vi "SmarAct micropositioner control.vi"() -> ()   [LabVIEW 2013]
uses:
  <vilib>/Utility/file.llb/Write To Spreadsheet File (DBL).vi
  <vilib>/DAQmx/configure/timing.llb/DAQmx Timing (Implicit).vi
  <vilib>/DAQmx/create/channels.llb/DAQmx Create Channel (CO-Pulse Generation-Frequency).vi
panel:
  in  "counter":tag="Dev1/ctr0" caption="计数器"
  out "frequency":dbl=1.0 format="%#_13g"
  out "duty cycle":dbl=0.5 caption="占空比" format="%.6f"
  in  "samples per channel":i32=5 caption="脉冲个数"
  in  "周期（ms）":dbl=1.0 format="%#_13g"
  in  "脉宽（us）":dbl=10.0 format="%#_13g"
  in  "initial delay":dbl format="%.6f"
  in  "X扫描步距":i16
  out "已完成行数":i32
  out "存储数据time,x,y":dbl[][](array[numeric])
  out "完成":bool
  out "error out":errorcluster
  in  "Y 初始位置":i32
  in  "X 初始位置":i32
  in  "X 返回速度":u32=50 min=1 max=4095000000
  out "error out 2":errorcluster
  out "XY 实时位置":u32[][](array[numeric])
  in  "Y 步距":i32
  in  "Y 扫描速度":u32=50 min=1 max=4095000000
  in  "Y 扫描范围":i32
  in  "X 扫描范围":i32
  in  "X 扫描速度":u32=50 min=1 max=4095000000
  in  "enabled 2":T1(ring)=enum."SA_SENSOR_POWERSAVE"
  in  "enabled":T2(ring)=enum."SA_HCM_ENABLED"
  in  "configuration":T3(ring)
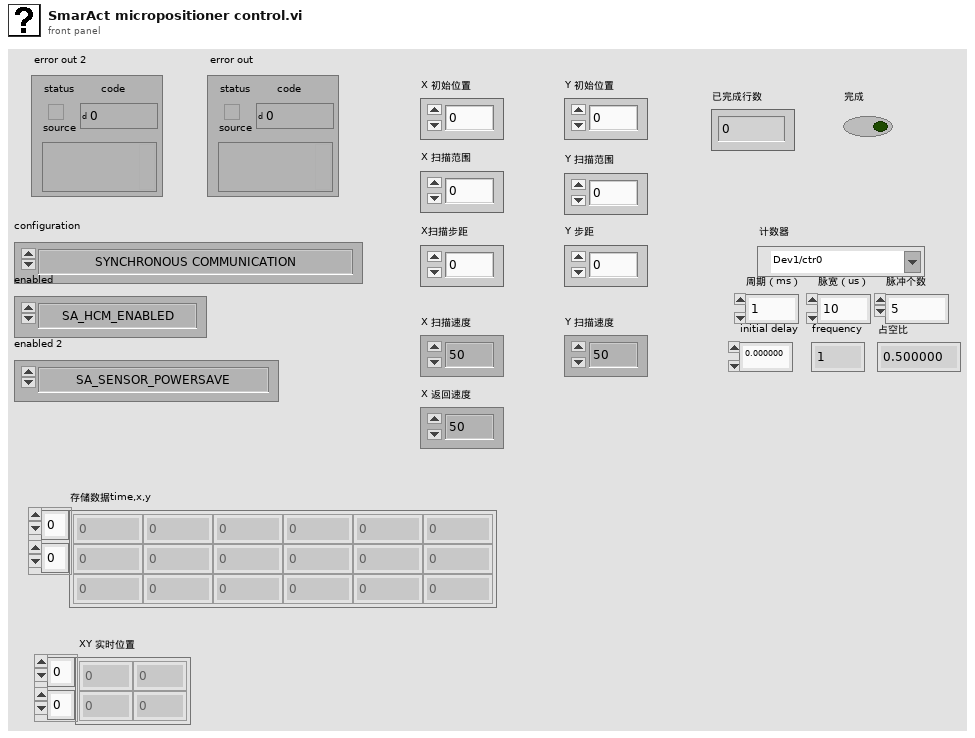
[diagram p1: front panel]
types:
  T1 = enum32{"SA_SENSOR_DISABLED", "SA_SENSOR_ENABLED", "SA_SENSOR_POWERSAVE"}
  T2 = enum32{"SA_HCM_DISABLED", "SA_HCM_ENABLED", "SA_HCM_CONTROLS_DISABLED"}
  T3 = enum32{"SYNCHRONOUS COMMUNICATION", "ASYNCHRONOUS COMMUNICATION", "SYNCHRONOUS COMMUNICATION WITH HARDWARE RESET", "ASYNCHRONOUS COMMUNICATION WITH HARDWARE RESET"}
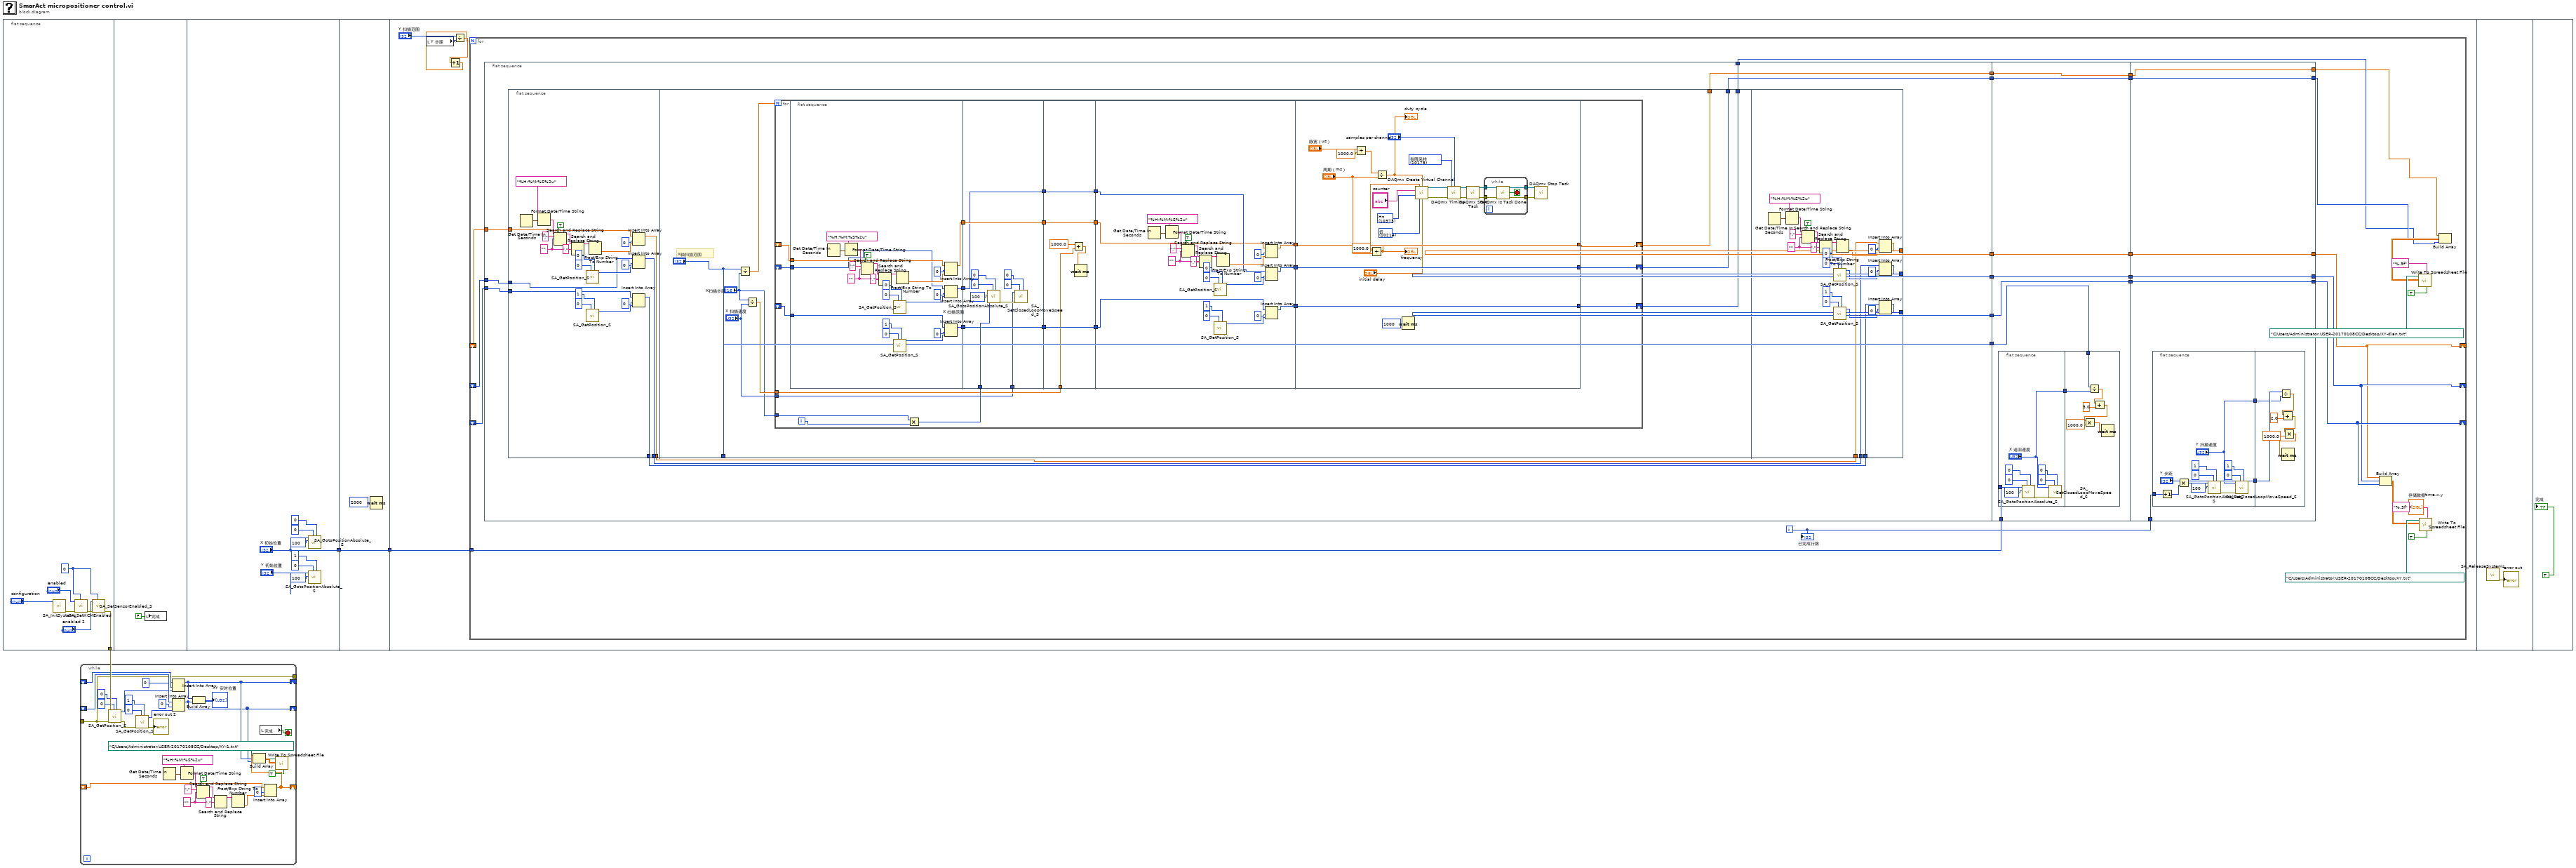
[diagram p0: block diagram]
diagram:
  n1 = flat-sequence {
    tunnel: [w5] -> w3
    tunnel: ["X 初始位置"] -> w1
    tunnel: [w20] -> w2
    tunnel: w1 -> [w20]
    tunnel: w2 -> [w24]
    frame #0 {
      w10 = u32 0 ("systemIndex")
      n2 = call <vilib>:"SA_InitSystems.vi"("configuration"="configuration") -> ("error out"=w4:errorcluster)  [unwired: 10 in]
      n3 = call <vilib>:"SA_SetHCMEnabled.vi"("systemIndex"=w10, "error in (no error)"=w4, "enabled"="enabled") -> ("error out"=w9:errorcluster)  [unwired: 8 in]
      n4 = call <vilib>:"SA_SetSensorEnabled_S.vi"("systemIndex"=w10, "error in (no error)"=w9, "enabled"="enabled 2") -> ("error out"=w5:errorcluster)  [unwired: 8 in]
    }
    frame #1 {
      n5 = local write "完成"(FALSE ("Finished")) -> ()
    }
    frame #2 {
      n6 = call <vilib>:"SA_GotoPositionAbsolute_S.vi"("channelIndex"=u32 0, "systemIndex"=u32 0, "holdTime"=u32 100, "position"="X 初始位置") -> ()  [unwired: 7 in, 1 out]
      n7 = call <vilib>:"SA_GotoPositionAbsolute_S.vi"("channelIndex"=u32 1, "systemIndex"=u32 0, "holdTime"=u32 100, "position"="Y 初始位置") -> ()  [unwired: 7 in, 1 out]
    }
    frame #3 {
      n8 = Wait (ms)(milliseconds to wait=u32 2000 ("等待时间（毫秒）")) -> ()  [unwired: 1 out]
    }
    frame #4 {
      n9 = local read "Y 步距"() -> (w26:i32)
      n10 = Divide(x="Y 扫描范围", y=w26) -> (x/y=w23:dbl)
      n11 = Increment(x=w23) -> (x+1=w22:dbl)
      n12 = for {
        N: w22 -> [_]
        tunnel: w24 -> [w55]
        shift-right: [w34] -> _
        shift-left: _ -> [w39]
        shift-right: [w35] -> _
        shift-left: _ -> [w38]
        shift-right: [w36] -> _
        shift-left: _ -> [w37]
        i -> [w56]
        n13 = flat-sequence {
          tunnel: [w69] -> w54
          tunnel: [w68] -> w52
          tunnel: [w67] -> w50
          tunnel: w37 -> [w66]
          tunnel: [w65] -> w44
          tunnel: [w64] -> w43
          tunnel: [w63] -> w40
          tunnel: [w62] -> w28
          tunnel: w39 -> [w58]
          tunnel: w38 -> [w57]
          tunnel: w55 -> [w255]
          tunnel: w54 -> [w254]
          tunnel: [w254] -> w53
          tunnel: w52 -> [w253]
          tunnel: [w253] -> w51
          tunnel: w50 -> [w252]
          tunnel: [w252] -> w49
          tunnel: w44 -> [w250]
          tunnel: w43 -> [w249]
          tunnel: [w249] -> w42
          tunnel: [w248] -> w41
          tunnel: w40 -> [w248]
          tunnel: w56 -> [w278]
          tunnel: w53 -> [w275]
          tunnel: w51 -> [w276]
          tunnel: [w275] -> w35
          tunnel: [w276] -> w36
          tunnel: w49 -> [w277]
          tunnel: [w277] -> w34
          tunnel: w42 -> [w272]
          tunnel: [w272] -> w27
          tunnel: w41 -> [w271]
          tunnel: [w271] -> w29
          frame #0 {
            n14 = flat-sequence {
              tunnel: w66 -> [w75]
              tunnel: [w74] -> w61
              tunnel: [w73] -> w60
              tunnel: [w72] -> w59
              tunnel: w58 -> [w71]
              tunnel: w57 -> [w70]
              tunnel: ["X 扫描范围"] -> w65
              tunnel: [w100] -> w64
              tunnel: [w99] -> w63
              tunnel: [w98] -> w62
              tunnel: [w247] -> w69
              tunnel: [w246] -> w68
              tunnel: [w226] -> w67
              tunnel: w61 -> [w225]
              tunnel: w60 -> [w224]
              tunnel: w59 -> [w223]
              frame #0 {
                w88 = "" ("替换字符串(\"\")")
                n15 = Get Date/Time In Seconds() -> (seconds since 1Jan1904=w83:timestamp)
                n16 = Format Date/Time String(time format string (%c)="%H:%M:%S%2u" ("时间格式字符串(%c)"), seconds (now)=w83) -> (date/time string=w84:string)  [unwired: 1 in]
                n17 = Search and Replace String(replace all?=TRUE ("替换全部？(F)"), input string=w84, search string=":" ("子字符串(\"\")"), replace string=w88) -> (result string=w90:string)  [unwired: 4 in, 3 out]
                n18 = Search and Replace String(input string=w90, search string="." ("搜索字符串"), replace string=w88) -> (result string=w87:string)  [unwired: 5 in, 3 out]
                n19 = call <vilib>:"SA_GetPosition_S.vi"("channelIndex"=u32 0, "systemIndex"=u32 0) -> ("position"=w77:i32)  [unwired: 8 in, 1 out]
                n20 = call <vilib>:"SA_GetPosition_S.vi"("channelIndex"=u32 1, "systemIndex"=u32 0) -> ("position"=w78:i32)  [unwired: 8 in, 1 out]
                n21 = Fract/Exp String To Number(string=w87) -> (number=w76:dbl)  [unwired: 3 in, 1 out]
                n22 = Insert Into Array(array=w71, index=0 ("索引"), new element=w76) -> (w74:dbl[])
                n23 = Insert Into Array(array=w70, index=0 ("索引"), new element=w77) -> (w73:i32[])
                n24 = Insert Into Array(array=w75, index=0 ("索引"), new element=w78) -> (w72:i32[])
              }
              frame #1 {
                # "X轴扫描范围"
                n25 = Divide(x="X 扫描范围", y="X扫描步距") -> (x/y=w101:dbl)
                n26 = Divide(x="X扫描步距", y="X 扫描速度") -> (x/y=w97:dbl)
                n27 = for {
                  N: w101 -> [_]
                  shift-right: [w103] -> w100
                  shift-left: _ -> [w104]
                  shift-right: [w115] -> w99
                  shift-left: _ -> [w113]
                  shift-right: [w114] -> w98
                  shift-left: _ -> [w112]
                  tunnel: w97 -> [w108]
                  tunnel: "X扫描步距" -> [w106]
                  tunnel: "X 扫描速度" -> [w105]
                  i -> [w107]
                  n28 = flat-sequence {
                    tunnel: [w131] -> w122
                    tunnel: [w130] -> w119
                    tunnel: [w129] -> w116
                    tunnel: w104 -> [w128]
                    tunnel: w113 -> [w127]
                    tunnel: w112 -> [w126]
                    tunnel: w125 -> [w155]
                    tunnel: [w154] -> w123
                    tunnel: w122 -> [w154]
                    tunnel: [w153] -> w120
                    tunnel: w119 -> [w153]
                    tunnel: [w152] -> w117
                    tunnel: w116 -> [w152]
                    tunnel: w105 -> [w151]
                    tunnel: [w165] -> w124
                    tunnel: w123 -> [w165]
                    tunnel: [w164] -> w121
                    tunnel: w120 -> [w164]
                    tunnel: [w163] -> w118
                    tunnel: w117 -> [w163]
                    tunnel: w108 -> [w162]
                    tunnel: w124 -> [w171]
                    tunnel: w121 -> [w173]
                    tunnel: w118 -> [w169]
                    tunnel: [w172] -> w111
                    tunnel: [w170] -> w110
                    tunnel: [w168] -> w109
                    tunnel: w111 -> [w217]
                    tunnel: w110 -> [w216]
                    tunnel: w109 -> [w215]
                    tunnel: [w217] -> w115
                    tunnel: [w216] -> w103
                    tunnel: [w215] -> w114
                    frame #0 {
                      w138 = "" ("替换字符串(\"\")")
                      n29 = Get Date/Time In Seconds() -> (seconds since 1Jan1904=w143:timestamp)
                      n30 = Format Date/Time String(time format string (%c)="%H:%M:%S%2u" ("时间格式字符串(%c)"), seconds (now)=w143) -> (date/time string=w142:string)  [unwired: 1 in]
                      n31 = Search and Replace String(replace all?=TRUE ("替换全部？(F)"), input string=w142, search string=":" ("子字符串(\"\")"), replace string=w138) -> (result string=w136:string)  [unwired: 4 in, 3 out]
                      n32 = Search and Replace String(input string=w136, search string="." ("搜索字符串"), replace string=w138) -> (result string=w139:string)  [unwired: 5 in, 3 out]
                      n33 = call <vilib>:"SA_GetPosition_S.vi"("channelIndex"=u32 0, "systemIndex"=u32 0) -> ("position"=w149:i32)  [unwired: 8 in, 1 out]
                      n34 = call <vilib>:"SA_GetPosition_S.vi"("channelIndex"=u32 1, "systemIndex"=u32 0) -> ("position"=w148:i32)  [unwired: 8 in, 1 out]
                      n35 = Fract/Exp String To Number(string=w139) -> (number=w150:dbl)  [unwired: 3 in, 1 out]
                      n36 = Insert Into Array(array=w128, index=0 ("索引"), new element=w150) -> (w131:dbl[])
                      n37 = Insert Into Array(array=w127, index=0 ("索引"), new element=w149) -> (w130:i32[])
                      n38 = Insert Into Array(array=w126, index=0 ("索引"), new element=w148) -> (w129:i32[])
                    }
                    frame #1 {
                      n39 = call <vilib>:"SA_GotoPositionAbsolute_S.vi"("channelIndex"=u32 0, "systemIndex"=u32 0, "holdTime"=u32 100, "position"=w155) -> ("error out"=w158:errorcluster)  [unwired: 7 in]
                      n40 = call <vilib>:"SA_SetClosedLoopMoveSpeed_S.vi"("channelIndex"=u32 0, "systemIndex"=u32 0, "error in (no error)"=w158, "speed"=w151) -> ()  [unwired: 7 in, 1 out]
                    }
                    frame #2 {
                      n41 = Add(x=1000.0, y=w162) -> (x+y=w166:dbl)
                      n42 = Wait (ms)(milliseconds to wait=w166) -> ()  [unwired: 1 out]
                    }
                    frame #3 {
                      w180 = "" ("替换字符串(\"\")")
                      n43 = Get Date/Time In Seconds() -> (seconds since 1Jan1904=w185:timestamp)
                      n44 = Format Date/Time String(time format string (%c)="%H:%M:%S%2u" ("时间格式字符串(%c)"), seconds (now)=w185) -> (date/time string=w184:string)  [unwired: 1 in]
                      n45 = Search and Replace String(replace all?=TRUE ("替换全部？(F)"), input string=w184, search string=":" ("子字符串(\"\")"), replace string=w180) -> (result string=w178:string)  [unwired: 4 in, 3 out]
                      n46 = Search and Replace String(input string=w178, search string="." ("搜索字符串"), replace string=w180) -> (result string=w181:string)  [unwired: 5 in, 3 out]
                      n47 = call <vilib>:"SA_GetPosition_S.vi"("channelIndex"=u32 0, "systemIndex"=u32 0) -> ("position"=w191:i32)  [unwired: 8 in, 1 out]
                      n48 = call <vilib>:"SA_GetPosition_S.vi"("channelIndex"=u32 1, "systemIndex"=u32 0) -> ("position"=w190:i32)  [unwired: 8 in, 1 out]
                      n49 = Fract/Exp String To Number(string=w181) -> (number=w192:dbl)  [unwired: 3 in, 1 out]
                      n50 = Insert Into Array(array=w171, index=0 ("索引"), new element=w192) -> (w170:dbl[])
                      n51 = Insert Into Array(array=w173, index=0 ("索引"), new element=w191) -> (w172:i32[])
                      n52 = Insert Into Array(array=w169, index=0 ("索引"), new element=w190) -> (w168:i32[])
                    }
                    frame #4 {
                      w200 = 10178 items=["有限采样"=10178, "连续采样"=10123, "硬件定时单点"=12522] ("sample mode")
                      w195 = 10214 items=["高"=10192, "低"=10214] ("idle state")
                      w194 = 10373 items=["Hz"=10373] ("units")
                      n53 = Divide(x="脉宽（us）", y=1000.0) -> (x/y=w212:dbl)
                      n54 = Divide(x=1000.0, y="周期（ms）") -> (x/y=w209:dbl)
                      "frequency" <- w209
                      n55 = Divide(x=w212, y="周期（ms）") -> (x/y=w214:dbl)
                      "duty cycle" <- w214
                      n56 = Wait (ms)(milliseconds to wait=u32 1000 ("等待时间（毫秒）")) -> ()  [unwired: 1 out]
                      n57 = call-poly <vilib>:"DAQmx Create Virtual Channel.vi"("frequency"=w209, "duty cycle"=w214, "counter"="counter", "units"=w194, "idle state"=w195, "initial delay"="initial delay") -> ("task out"=w198:refnum<k21>, "error out"=w199:errorcluster)  [unwired: 8 in]
                      n58 = call-poly <vilib>:"DAQmx Timing.vi"("task/channels in"=w198, "sample mode"=w200, "samples per channel"="samples per channel", "error in"=w199) -> ("task out"=w202:refnum<k21>, "error out"=w203:errorcluster)  [unwired: 10 in]
                      n59 = call <vilib>:"DAQmx Start Task.vi"("task/channels in"=w202, "error in"=w203) -> ("task out"=w204:refnum<k21>, "error out"=w205:errorcluster)  [unwired: 12 in]
                      n60 = while {
                        tunnel: w204 -> [w222]
                        tunnel: w205 -> [w221]
                        tunnel: [w219] -> w206
                        tunnel: [w218] -> w207
                        stop <- w220 stop-if-true
                        n61 = call <vilib>:"DAQmx Is Task Done.vi"("task/channels in"=w222, "error in"=w221) -> ("task out"=w219:refnum<k21>, "task done?"=w220:bool, "error out"=w218:errorcluster)  [unwired: 11 in]
                      }
                      n62 = call <vilib>:"DAQmx Stop Task.vi"("task/channels in"=w206, "error in"=w207) -> ()  [unwired: 12 in, 2 out]
                    }
                  }
                  n63 = Multiply(x=w106, y=w107) -> (x*y=w125:i32)
                }
              }
              frame #2 {
                w238 = "" ("替换字符串(\"\")")
                n64 = Get Date/Time In Seconds() -> (seconds since 1Jan1904=w233:timestamp)
                n65 = Format Date/Time String(time format string (%c)="%H:%M:%S%2u" ("时间格式字符串(%c)"), seconds (now)=w233) -> (date/time string=w234:string)  [unwired: 1 in]
                n66 = Search and Replace String(replace all?=TRUE ("替换全部？(F)"), input string=w234, search string=":" ("子字符串(\"\")"), replace string=w238) -> (result string=w240:string)  [unwired: 4 in, 3 out]
                n67 = Search and Replace String(input string=w240, search string="." ("搜索字符串"), replace string=w238) -> (result string=w237:string)  [unwired: 5 in, 3 out]
                n68 = call <vilib>:"SA_GetPosition_S.vi"("channelIndex"=u32 0, "systemIndex"=u32 0) -> ("position"=w227:i32)  [unwired: 8 in, 1 out]
                n69 = call <vilib>:"SA_GetPosition_S.vi"("channelIndex"=u32 1, "systemIndex"=u32 0) -> ("position"=w228:i32)  [unwired: 8 in, 1 out]
                n70 = Fract/Exp String To Number(string=w237) -> (number=w231:dbl)  [unwired: 3 in, 1 out]
                n71 = Insert Into Array(array=w225, index=0 ("索引"), new element=w231) -> (w226:dbl[])
                n72 = Insert Into Array(array=w224, index=0 ("索引"), new element=w227) -> (w247:i32[])
                n73 = Insert Into Array(array=w223, index=0 ("索引"), new element=w228) -> (w246:i32[])
              }
            }
          }
          frame #1 {
            n74 = flat-sequence {
              tunnel: w255 -> [w257]
              tunnel: ["X 返回速度"] -> w251
              tunnel: w251 -> [w270]
              tunnel: w250 -> [w267]
              frame #0 {
                n75 = call <vilib>:"SA_GotoPositionAbsolute_S.vi"("channelIndex"=u32 0, "systemIndex"=u32 0, "holdTime"=u32 100, "position"=w257) -> ("error out"=w261:errorcluster)  [unwired: 7 in]
                n76 = call <vilib>:"SA_SetClosedLoopMoveSpeed_S.vi"("channelIndex"=u32 0, "systemIndex"=u32 0, "error in (no error)"=w261, "speed"="X 返回速度") -> ()  [unwired: 7 in, 1 out]
              }
              frame #1 {
                n77 = Divide(x=w267, y=w270) -> (x/y=w269:dbl)
                n78 = Add(x=w269, y=3.0) -> (x+y=w266:dbl)
                n79 = Multiply(x=w266, y=1000.0) -> (x*y=w265:dbl)
                n80 = Wait (ms)(milliseconds to wait=w265) -> ()  [unwired: 1 out]
              }
            }
          }
          frame #2 {
            n81 = flat-sequence {
              tunnel: w278 -> [w282]
              tunnel: ["Y 步距"] -> w274
              tunnel: ["Y 扫描速度"] -> w273
              tunnel: w274 -> [w296]
              tunnel: w273 -> [w295]
              frame #0 {
                n82 = Increment(x=w282) -> (x+1=w283:i32)
                n83 = Multiply(x="Y 步距", y=w283) -> (x*y=w284:i32)
                n84 = call <vilib>:"SA_GotoPositionAbsolute_S.vi"("channelIndex"=u32 1, "systemIndex"=u32 0, "holdTime"=u32 100, "position"=w284) -> ("error out"=w287:errorcluster)  [unwired: 7 in]
                n85 = call <vilib>:"SA_SetClosedLoopMoveSpeed_S.vi"("channelIndex"=u32 1, "systemIndex"=u32 0, "error in (no error)"=w287, "speed"="Y 扫描速度") -> ()  [unwired: 7 in, 1 out]
              }
              frame #1 {
                n86 = Divide(x=w296, y=w295) -> (x/y=w294:dbl)
                n87 = Add(x=w294, y=2.0) -> (x+y=w290:dbl)
                n88 = Multiply(x=w290, y=1000.0) -> (x*y=w292:dbl)
                n89 = Wait (ms)(milliseconds to wait=w292) -> ()  [unwired: 1 out]
              }
            }
          }
        }
        n90 = Build Array(w34, w35, w36) -> (w45:dbl[][])
        n91 = call-poly <vilib>:"Write To Spreadsheet File.vi"("transpose? (no:F)"=TRUE, "format (%.3f)"="%.3f" ("format (%d)"), "2D data"=w45, "file path (dialog if empty)"=path "C:/Users/Administrator.USER-20170108CC/Desktop/XY.txt") -> ()  [unwired: 4 in, 1 out]
        n92 = Build Array(w27, w29, w28) -> (w30:dbl[][])
        n93 = call-poly <vilib>:"Write To Spreadsheet File.vi"("transpose? (no:F)"=TRUE, "format (%.3f)"="%.3f" ("format (%d)"), "2D data"=w30, "file path (dialog if empty)"=path "C:/Users/Administrator.USER-20170108CC/Desktop/XY-dian.txt") -> ()  [unwired: 4 in, 1 out]
        "已完成行数" <- w56
      }
    }
    frame #5 {
      n94 = call <vilib>:"SA_ReleaseSystems.vi"() -> ("error out"=→"error out":errorcluster)  [unwired: 11 in]
    }
    frame #6 {
      "完成" <- TRUE ("Finished")
    }
  }
  n95 = while {
    tunnel: [w318] -> _
    shift-right: [w303] -> _
    shift-left: _ -> [w331]
    shift-right: [w302] -> _
    shift-left: _ -> [w330]
    tunnel: w3 -> [w318]
    shift-right: [w304] -> _
    shift-left: _ -> [w305]
    stop <- w317 stop-if-true
    w314 = "" ("替换字符串(\"\")")
    n96 = call <vilib>:"SA_GetPosition_S.vi"("channelIndex"=u32 0, "systemIndex"=u32 0, "error in (no error)"=w318) -> ("error out"=w323:errorcluster, "position"=w324:i32)  [unwired: 7 in]
    n97 = call <vilib>:"SA_GetPosition_S.vi"("channelIndex"=u32 1, "systemIndex"=u32 0, "error in (no error)"=w323) -> ("error out"=→"error out 2":errorcluster, "position"=w319:i32)  [unwired: 7 in]
    n98 = Get Date/Time In Seconds() -> (seconds since 1Jan1904=w309:timestamp)
    n99 = Insert Into Array(array=w331, index=0 ("索引"), new element=w324) -> (w303:i32[])
    n100 = Insert Into Array(array=w330, index=0 ("索引"), new element=w319) -> (w302:i32[])
    n101 = Format Date/Time String(time format string (%c)="%H:%M:%S%2u" ("时间格式字符串(%c)"), seconds (now)=w309) -> (date/time string=w310:string)  [unwired: 1 in]
    n102 = Build Array(w303, w302) -> (→"XY 实时位置":i32[][])
    n103 = Search and Replace String(replace all?=TRUE ("替换全部？(F)"), input string=w310, search string=":" ("子字符串(\"\")"), replace string=w314) -> (result string=w316:string)  [unwired: 4 in, 3 out]
    n104 = Search and Replace String(input string=w316, search string="." ("搜索字符串"), replace string=w314) -> (result string=w313:string)  [unwired: 5 in, 3 out]
    n105 = Fract/Exp String To Number(string=w313) -> (number=w307:dbl)  [unwired: 3 in, 1 out]
    n106 = local read "完成"() -> (w317:bool)
    n107 = Insert Into Array(array=w305, index=0 ("索引"), new element=w307) -> (w304:dbl[])
    n108 = Build Array(w304, w303, w302) -> (w301:dbl[][])
    n109 = call-poly <vilib>:"Write To Spreadsheet File.vi"("transpose? (no:F)"=TRUE, "2D data"=w301, "file path (dialog if empty)"=path "C:/Users/Administrator.USER-20170108CC/Desktop/XY-1.txt") -> ()  [unwired: 5 in, 1 out]
  }
